vi "PD23X Test.vi"() -> ()   [LabVIEW 2019]
uses:
  <instrlib>/_KELLER RS485 Library/Public/Type Definitions/Information.ctl
  <instrlib>/_KELLER RS485 Library/Public/Type Definitions/Status byte.ctl
  <instrlib>/_KELLER RS485 Library/Public/Type Definitions/Channel.ctl
  <instrlib>/_KELLER RS485 Library/Public/Type Definitions/Baud Rate.ctl
  <instrlib>/_KELLER RS485 Library/KELLER RS485 Library.lvlib
panel:
  out "number":u32
  out "Serial number out":u32
  out "Configuration out dec":u8 format="%0d"
  out "Configuration out hex":u8 format="%0x"
  out "Status byte":u8
  in  "Read Configuration Number (0)":u8
  out "Configuration out":u8 format="%08b"
  in  "Channel (P1)":T1=enum."P1"
  out "Status (STAT)":T2
  out "Value as Single":sgl format="%#.6f"
  out "Firmware Version out":string
  out "Information out":T3
  # "76543210"
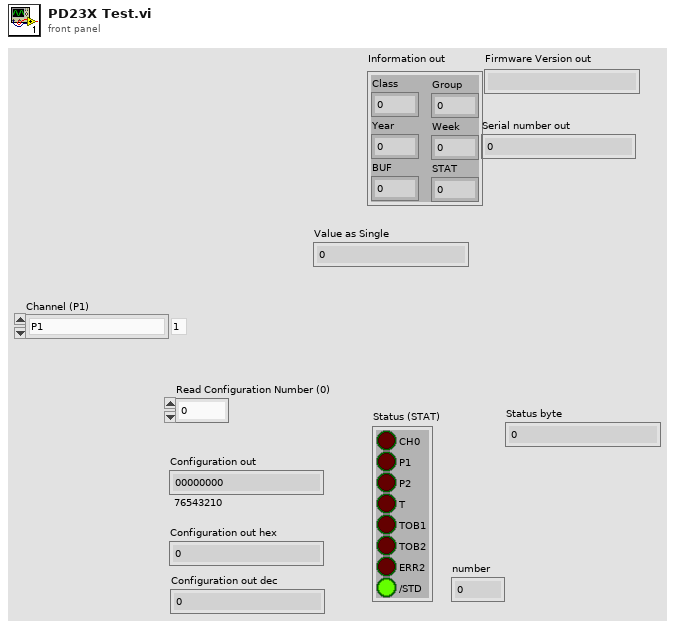
[diagram p1: front panel]
types:
  T1 = typedef "KELLER RS485 Library.lvlib/Channel.ctl" = enum16{"CH0", "P1", "P2", "T", "TOB1", "TOB2", "TE", "CH7", "CH8", "CH9", "ConTc", "ConRaw", "CH12"}
  T2 = typedef "KELLER RS485 Library.lvlib/Status byte.ctl" = cluster{"CH0":bool, "P1":bool, "P2":bool, "T":bool, "TOB1":bool, "TOB2":bool, "ERR2":bool, "/STD":bool}
  T3 = typedef "KELLER RS485 Library.lvlib/Information.ctl" = cluster{"Class":u8, "Group":u8, "Year":u8, "Week":u8, "BUF":u8, "STAT":u8}
  T4 = typedef "KELLER RS485 Library.lvlib/Baud Rate.ctl" = enum16{"9600bd", "115200bd"}
  T5 = typedef "KELLER RS485 Library.lvlib/Bus.ctl" = cluster{"VISA":refnum<visa-resource-name>, "Baud Rate ":T4, "Timeout":u32, "Echo?":bool, "Wait before transmit":u32}
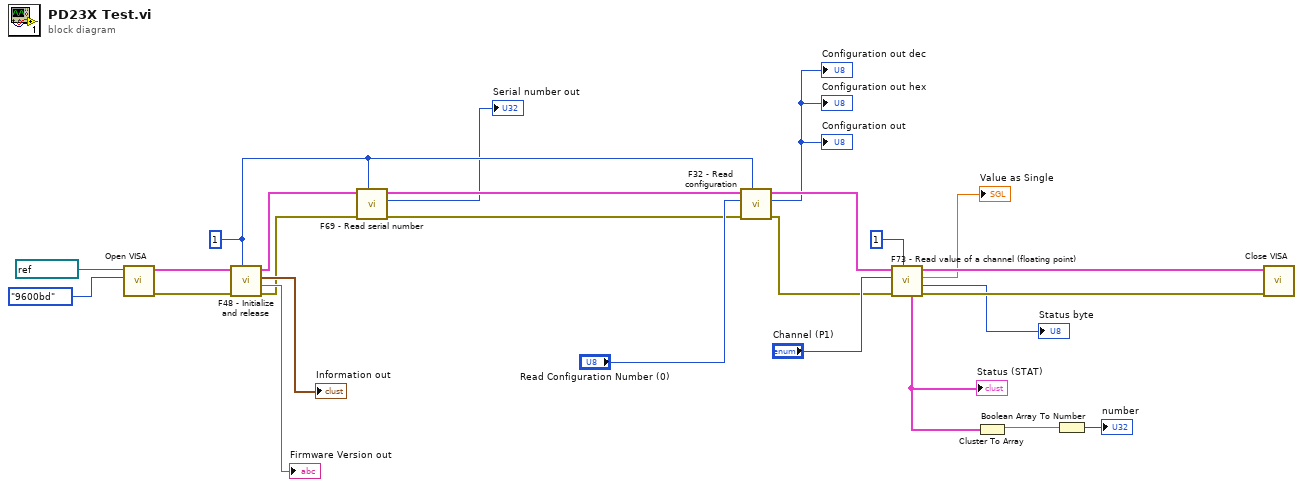
[diagram p0: block diagram]
diagram:
  w7 = u8 1 ("Address (250)")
  n1 = call <instrlib>:"Open VISA.vi"("Baud Rate (9600bd)"=Baud_Rate."9600bd", "VISA resource name"=refnum<visa-resource-name> "CH340") -> ("error out"=w17:errorcluster, "Bus out"=w18:T5)  [unwired: 8 in]
  n2 = call <instrlib>:"F48 - Initialize and release.vi"("Address (250)"=w7, "error in (no error)"=w17, "Bus in"=w18) -> ("error out"=w8:errorcluster, "Firmware Version out"=→"Firmware Version out":string, "Information out"=→"Information out":T3, "Bus out"=w9:T5)  [unwired: 5 in]
  n3 = call <instrlib>:"F69 - Read serial number.vi"("Address (250)"=w7, "error in (no error)"=w8, "Bus in"=w9) -> ("error out"=w5:errorcluster, "Serial number out"=→"Serial number out":u32, "Bus out"=w6:T5)  [unwired: 6 in]
  n4 = call <instrlib>:"F32 - Read configuration.vi"("Address (250)"=w7, "error in (no error)"=w5, "Configuration Number (0)"="Read Configuration Number (0)", "Bus in"=w6) -> ("error out"=w12:errorcluster, "Configuration out"=→"Configuration out" →"Configuration out hex" →"Configuration out dec":u8, "Bus out"=w13:T5)  [unwired: 5 in]
  n5 = call <instrlib>:"F73 - Read value of a channel (floating point).vi"("Address (250)"=u8 1, "error in (no error)"=w12, "Channel (P1)"="Channel (P1)", "Bus in"=w13) -> ("error out"=w22:errorcluster, "Status byte"=→"Status byte":u8, "Value as Single"=→"Value as Single":sgl, "Bus out"=w23:T5, "Status (STAT)"=w3:T2)  [unwired: 3 in]
  "Status (STAT)" <- w3
  n6 = Cluster To Array(cluster=w3) -> (array=w2:bool[])
  n7 = Boolean Array To Number(Boolean array=w2) -> (number=→"number":u32)
  n8 = call <instrlib>:"Close VISA.vi"("error in (no error)"=w22, "Bus in"=w23) -> ()  [unwired: 9 in, 1 out]
